vi "Main_09a.vi"() -> ()   [LabVIEW 2020]
uses:
  Point.ctl
panel:
  out "Tail Positon count":i32
  in  "Puzzle":string="R 1\nD 1\nL 1\nD 1\nR 2\nL 1\nU 2\nD 1\nU 2\nL 1\nU 1\nL 2\nD 1\nU 2\nL 1\nR 1\nD 1\nL 2\nD 2\nL 2\nR 1\nL 2\nU 2\nR 2\nL 2\nU 2\nL 1\nD 1\nL 2\nU 1\nR 1\nD 2\nL 2\nU 1\nR 1\nD 1\nU 2\nL 1\nD 2\nU 1\nD 1\nR 2\nD 1\nL 2\nD 1\nL 1\nR 1\nD 2\nL 1\nR 2\nD 2\nU 2\nR 2\nD 2\nR 2\nL 2\nD 2\nL 2\nD 1\nU 2\nR 1\nD 2\nL 2\nR 2\nL 1\nD 1\nU 2\nD 1\nR 2\nU 2\nR 2\nD 1\nL 1\nU 2\nD 1\nU 1\nD 2\nU 1\nR 1\nU 2\nD 1\nL 2\nU 1\nL 2\nD 2\nR 1\nU 2\nL 1\nD 2\nR 1\nU 1\nD 1\nL 2\nU 1\nR 1\nD 2\nU 2\nL 1\nU 2\nD 2\nR 1\nU 2\nR 1\nU 2\nR 1\nD 2\nU 1\nD 2\nL 2\nD 2\nL 2\nD 2\nR 1\nU 1\nD 3\nU 1\nR 2\nU 3\nD 1\nU 2\nD 2\nU 2\nD 1\nU 2\nR 2\nL 2\nU 1\nL 3\nD 1\nR 3\nD 3\nR 2\nL 1\nU 3\nD 1\nU 2\nR 2\nD 1\nR 3\nD 2\nR 3\nD 1\nU 3\nL 3\nR 2\nU 3\nL 3\nU 2\nL 3\nD 1\nR 3\nU 3\nR 2\nD 1\nU 3\nR 3\nD 1\nL 2\nD 2\nL 2\nD 3\nR 2\nU 3\nL 3\nD 2\nU 3\nL 2\nU 3\nD 1\nL 1\nD 3\nR 1\nD 3\nU 1\nL 3\nU 1\nD 2\nU 1\nD 1\nU 2\nD 3\nL 1\nU 1\nR 1\nU 3\nD 3\nR 1\nL 2\nR 3\nL 3\nU 1\nD 2\nR 2\nU 2\nD 3\nU 2\nD 3\nL 1\nR 3\nD 3\nR 2\nU 3\nD 3\nL 2\nR 3\nD 3\nR 2\nL 1\nR 3\nD 2\nR 1\nD 3\nL 1\nU 1\nD 2\nR 1\nD 1\nL 1\nR 2\nL 1\nU 1\nL 2\nD 2\nL 2\nD 1\nL 2\nU 3\nD 1\nR 3\nL 2\nR 1\nL 2\nR 3\nU 2\nL 4\nR 3\nL 1\nR 2\nD 2\nL 4\nU 3\nL 1\nD 1\nL 3\nU 2\nL 3\nU 2\nL 1\nR 2\nL 3\nU 1\nD 2\nR 1\nL 4\nR 4\nL 4\nU 2\nD 2\nR 2\nL 2\nU 2\nR 1\nD 3\nL 4\nR 2\nU 1\nL 4\nR 1\nL 1\nD 4\nR 3\nD 1\nR 2\nL 2\nR 3\nL 1\nU 1\nD 3\nU 2\nR 1\nL 1\nD 3\nR 2\nU 2\nR 3\nU 2\nD 1\nR 4\nU 4\nD 3\nU 3\nR 2\nU 1\nL 1\nU 4\nD 1\nR 4\nD 4\nL 3\nU 4\nR 4\nL 1\nR 1\nU 2\nR 4\nD 2\nR 1\nU 2\nL 1\nD 1\nL 3\nR 3\nL 3\nD 3\nL 4\nD 2\nU 2\nD 3\nR 1\nU 1\nD 3\nU 1\nR 3\nD 2\nL 3\nR 2\nD 1\nL 3\nD 3\nU 3\nD 4\nL 2\nU 3\nD 5\nL 2\nD 2\nR 2\nL 3\nD 5\nU 4\nR 1\nD 5\nR 1\nD 1\nL 2\nR 4\nU 2\nD 3\nR 5\nL 2\nR 2\nD 1\nR 2\nU 5\nL 4\nU 5\nD 1\nL 2\nU 2\nR 2\nD 4\nU 3\nL 2\nD 1\nU 4\nL 4\nD 3\nL 3\nD 3\nR 1\nU 1\nR 1\nU 1\nR 2\nD 3\nR 5\nU 1\nD 2\nL 5\nU 5\nL 4\nD 4\nU 4\nL 1\nR 5\nU 2\nL 3\nU 2\nD 3\nL 5\nD 5\nL 2\nU 2\nD 4\nU 3\nD 3\nL 1\nD 2\nR 2\nD 1\nR 4\nL 3\nD 1\nU 4\nL 1\nR 2\nL 4\nD 5\nR 3\nD 1\nL 5\nD 5\nU 3\nR 2\nD 4\nL 2\nR 2\nD 3\nR 3\nU 2\nR 5\nU 4\nR 3\nL 1\nD 2\nU 1\nL 1\nR 2\nU 4\nD 4\nL 1\nR 1\nU 4\nL 3\nU 5\nR 3\nL 4\nD 3\nU 1\nR 4\nU 1\nL 1\nU 3\nR 4\nL 5\nD 1\nU 4\nR 5\nL 1\nR 4\nD 2\nL 6\nD 5\nU 5\nL 5\nR 6\nD 1\nU 2\nR 1\nU 4\nD 6\nL 6\nD 6\nU 6\nD 4\nU 4\nD 1\nU 3\nL 5\nD 6\nR 1\nL 1\nD 2\nL 4\nD 4\nL 4\nR 4\nU 2\nL 3\nD 4\nR 3\nD 4\nU 5\nR 4\nU 1\nR 6\nL 3\nR 2\nU 1\nL 1\nR 2\nD 3\nR 6\nD 6\nU 1\nD 3\nU 4\nD 5\nL 5\nU 3\nD 6\nL 5\nR 5\nU 1\nR 4\nD 2\nL 2\nR 4\nL 5\nR 4\nL 3\nD 5\nR 6\nL 6\nU 1\nR 5\nU 6\nD 2\nR 2\nD 1\nL 6\nU 4\nL 1\nR 5\nL 1\nR 2\nD 1\nL 4\nU 4\nL 1\nR 3\nU 5\nL 2\nD 6\nU 5\nR 6\nD 6\nU 3\nL 3\nU 3\nL 4\nD 5\nU 2\nD 4\nU 5\nR 6\nU 5\nD 2\nU 6\nD 3\nL 3\nD 6\nL 5\nR 2\nD 6\nR 7\nD 3\nL 7\nD 3\nU 2\nR 7\nU 2\nL 6\nR 7\nD 3\nR 7\nU 5\nR 7\nL 5\nR 7\nL 7\nU 4\nD 4\nU 1\nD 3\nU 1\nD 5\nR 3\nU 1\nD 2\nU 1\nL 4\nU 2\nL 6\nD 7\nU 1\nD 4\nU 6\nL 4\nR 4\nD 4\nR 6\nD 7\nR 1\nD 7\nL 4\nR 4\nL 1\nU 1\nR 6\nL 7\nD 7\nL 5\nU 7\nD 3\nL 6\nD 6\nU 4\nR 1\nL 2\nD 4\nR 3\nL 1\nR 7\nD 1\nL 2\nU 1\nD 2\nR 1\nU 3\nD 4\nL 3\nU 6\nL 4\nR 2\nL 1\nU 6\nD 1\nR 5\nU 2\nD 2\nL 7\nU 2\nR 5\nD 2\nR 4\nD 4\nR 3\nL 2\nR 3\nU 7\nL 5\nR 7\nU 2\nL 7\nD 3\nU 6\nD 4\nU 4\nD 6\nU 3\nL 6\nR 4\nD 2\nR 4\nD 2\nR 3\nL 5\nD 1\nU 7\nD 4\nL 4\nU 2\nD 2\nU 7\nL 5\nR 6\nU 8\nL 7\nD 2\nU 1\nR 6\nD 4\nL 4\nR 7\nD 1\nL 6\nD 7\nR 7\nU 3\nL 6\nU 1\nL 8\nD 6\nU 8\nL 7\nU 5\nD 8\nL 2\nD 3\nL 8\nU 1\nD 5\nL 4\nR 6\nD 8\nL 6\nU 5\nR 3\nU 7\nR 6\nU 3\nL 3\nD 4\nR 4\nL 2\nR 6\nD 3\nR 3\nL 8\nU 2\nD 6\nU 3\nD 8\nU 6\nD 4\nU 8\nR 7\nD 2\nU 6\nD 6\nR 1\nU 3\nD 3\nR 1\nU 3\nR 1\nD 7\nL 8\nR 8\nU 7\nR 3\nL 8\nU 2\nL 8\nD 4\nU 4\nR 1\nD 3\nR 4\nU 3\nL 7\nU 2\nR 7\nD 2\nU 4\nD 3\nL 8\nD 5\nL 3\nU 4\nD 6\nL 5\nD 2\nU 1\nR 6\nL 4\nR 6\nU 5\nR 8\nU 8\nD 7\nL 5\nD 2\nL 8\nU 2\nD 1\nR 1\nL 7\nU 4\nR 2\nU 7\nD 6\nR 6\nL 5\nU 8\nD 7\nR 8\nL 8\nD 6\nU 6\nR 1\nD 5\nL 7\nR 8\nL 4\nD 3\nL 2\nU 5\nR 9\nL 8\nD 8\nL 2\nR 4\nL 7\nR 5\nL 1\nR 8\nD 8\nL 4\nU 2\nD 7\nL 7\nD 6\nR 8\nL 3\nD 7\nU 1\nR 6\nD 6\nU 6\nL 9\nD 1\nR 7\nL 5\nR 5\nU 5\nD 4\nL 8\nU 4\nD 8\nR 4\nD 6\nU 3\nD 7\nL 5\nD 6\nR 9\nU 4\nR 6\nL 3\nU 4\nD 9\nL 7\nR 5\nD 9\nL 6\nU 7\nL 7\nR 4\nD 5\nR 7\nL 5\nR 3\nU 8\nL 6\nU 5\nL 9\nR 8\nU 4\nD 2\nL 4\nD 7\nR 7\nD 4\nL 4\nU 2\nL 3\nR 1\nD 3\nU 6\nR 1\nU 8\nR 2\nL 4\nD 3\nL 5\nU 4\nR 7\nL 2\nR 7\nL 9\nD 9\nU 5\nL 4\nU 1\nD 1\nU 6\nD 1\nL 6\nD 7\nU 5\nD 9\nR 9\nD 5\nU 9\nL 3\nR 5\nD 10\nR 1\nU 7\nD 6\nL 3\nU 5\nR 1\nD 5\nR 8\nU 3\nL 1\nD 2\nR 1\nL 6\nR 8\nD 9\nU 9\nD 4\nR 1\nU 8\nL 5\nU 4\nD 7\nL 1\nR 4\nL 6\nD 4\nR 5\nD 1\nR 10\nD 5\nR 7\nU 6\nR 5\nU 2\nL 8\nR 1\nU 3\nL 5\nU 4\nL 3\nD 3\nU 6\nD 10\nL 3\nD 7\nL 5\nD 4\nU 6\nR 9\nU 5\nD 5\nR 2\nL 7\nU 8\nD 5\nR 9\nL 6\nR 8\nU 9\nL 4\nR 10\nD 10\nL 9\nR 8\nL 4\nR 5\nL 9\nD 1\nL 3\nR 9\nU 2\nL 5\nR 2\nU 1\nR 4\nD 10\nU 3\nD 8\nL 9\nD 8\nL 5\nD 4\nU 2\nL 8\nR 5\nU 4\nD 1\nL 4\nU 7\nD 9\nR 3\nD 7\nR 9\nL 6\nR 6\nU 8\nL 10\nU 5\nD 4\nR 5\nL 6\nD 7\nL 10\nR 1\nL 9\nU 6\nD 9\nR 7\nL 7\nD 6\nU 6\nR 1\nD 7\nL 1\nR 9\nD 9\nR 3\nL 5\nD 4\nR 3\nL 5\nD 11\nU 1\nR 6\nD 8\nR 4\nD 3\nR 9\nU 3\nD 8\nU 7\nR 2\nU 10\nR 4\nL 4\nD 10\nR 8\nU 11\nR 7\nD 7\nR 9\nD 11\nU 6\nR 7\nD 10\nL 4\nD 5\nL 7\nD 3\nL 4\nD 4\nU 4\nR 3\nL 9\nD 4\nL 8\nU 5\nR 7\nL 2\nD 4\nR 11\nU 10\nD 3\nR 8\nD 3\nR 10\nL 8\nU 6\nR 4\nD 10\nR 7\nD 3\nR 2\nU 1\nD 5\nL 8\nU 2\nR 1\nU 8\nR 11\nL 3\nU 10\nL 5\nD 3\nL 6\nU 10\nL 11\nD 4\nL 5\nD 1\nL 4\nD 1\nL 3\nR 7\nU 7\nR 4\nL 1\nU 10\nD 11\nL 1\nR 1\nU 9\nD 6\nL 9\nD 1\nL 4\nD 11\nL 5\nU 2\nL 5\nD 8\nU 10\nD 5\nU 10\nL 8\nR 11\nD 10\nU 11\nR 4\nU 6\nD 11\nR 1\nL 4\nU 12\nL 8\nU 12\nD 4\nL 7\nU 7\nL 8\nD 3\nU 1\nL 12\nD 5\nU 3\nD 6\nR 7\nU 1\nD 12\nR 6\nU 3\nD 3\nR 12\nU 5\nR 3\nU 8\nL 6\nR 6\nU 3\nL 4\nD 8\nL 5\nD 12\nU 1\nL 9\nR 4\nL 1\nD 6\nU 9\nL 5\nR 3\nL 9\nD 8\nR 6\nD 3\nU 6\nL 1\nD 7\nU 5\nD 1\nL 11\nR 7\nD 11\nL 3\nU 6\nR 9\nD 12\nR 11\nL 5\nR 8\nL 2\nU 10\nR 6\nU 10\nL 9\nU 1\nL 1\nR 8\nL 7\nR 3\nU 4\nL 3\nR 8\nL 9\nR 11\nL 9\nD 11\nU 1\nL 12\nR 6\nL 3\nR 3\nD 12\nU 9\nL 9\nD 8\nR 4\nL 7\nR 1\nU 2\nR 4\nU 4\nR 11\nU 7\nD 11\nU 3\nD 6\nU 7\nL 2\nD 4\nU 9\nR 3\nL 8\nR 9\nL 4\nR 5\nL 7\nD 3\nR 8\nL 6\nU 10\nR 3\nL 6\nD 8\nU 3\nD 9\nL 1\nU 13\nR 12\nL 13\nR 2\nU 8\nR 1\nD 11\nR 5\nL 4\nU 5\nL 3\nD 13\nU 2\nD 1\nU 2\nL 9\nD 3\nR 6\nU 13\nL 3\nU 5\nR 2\nD 2\nL 5\nU 4\nR 6\nD 1\nU 9\nL 7\nR 11\nU 10\nD 12\nR 10\nU 7\nR 5\nL 2\nR 13\nL 13\nD 3\nR 7\nU 1\nL 1\nD 2\nL 9\nU 12\nD 7\nU 13\nL 12\nU 13\nD 7\nU 7\nD 8\nL 2\nU 6\nD 2\nU 6\nL 8\nU 4\nD 11\nU 11\nL 11\nR 10\nL 10\nR 6\nD 13\nU 2\nL 7\nU 8\nD 1\nR 6\nL 7\nR 9\nL 8\nR 9\nL 6\nR 7\nD 12\nR 11\nL 8\nR 1\nD 5\nR 5\nL 10\nU 6\nL 8\nD 9\nL 5\nU 4\nD 12\nU 8\nL 13\nU 6\nD 10\nR 5\nL 13\nD 7\nL 13\nR 5\nL 10\nD 13\nL 9\nR 3\nD 8\nU 9\nD 10\nU 10\nD 7\nL 5\nR 5\nD 9\nL 7\nR 10\nD 13\nR 1\nU 2\nR 6\nU 14\nR 10\nD 6\nU 13\nD 14\nU 5\nD 1\nU 8\nR 4\nU 9\nR 13\nL 4\nD 2\nR 8\nU 2\nD 12\nU 3\nR 6\nU 6\nD 11\nR 7\nL 12\nR 9\nU 7\nD 1\nR 14\nL 11\nU 4\nD 13\nU 5\nL 7\nR 14\nL 1\nU 6\nD 3\nL 1\nU 13\nD 8\nU 14\nD 5\nU 14\nL 1\nR 1\nD 5\nU 7\nL 8\nR 6\nU 1\nD 2\nR 14\nU 13\nL 10\nU 8\nD 13\nU 6\nR 2\nD 4\nR 6\nU 7\nD 10\nL 6\nU 5\nL 3\nD 9\nU 13\nD 8\nU 3\nR 3\nL 12\nD 5\nR 8\nU 7\nR 11\nU 6\nD 7\nR 13\nU 1\nD 9\nU 10\nD 3\nL 5\nR 12\nL 4\nD 13\nR 7\nD 12\nR 11\nD 9\nR 5\nU 13\nR 3\nD 4\nU 10\nR 3\nU 6\nL 4\nR 1\nU 4\nL 9\nD 11\nU 5\nD 3\nU 13\nD 1\nL 1\nD 13\nL 2\nR 9\nL 4\nR 2\nU 9\nD 9\nU 12\nL 14\nR 2\nL 9\nR 5\nU 2\nD 3\nR 13\nU 5\nD 1\nU 15\nR 6\nD 14\nR 8\nL 9\nD 14\nL 6\nR 8\nU 14\nR 11\nL 3\nD 15\nU 5\nR 1\nL 7\nR 12\nD 1\nR 4\nD 13\nU 9\nD 2\nL 3\nU 10\nR 10\nD 2\nR 6\nU 13\nD 7\nR 5\nU 5\nL 12\nU 6\nR 1\nL 7\nU 9\nD 15\nL 8\nU 9\nL 5\nR 3\nL 9\nU 6\nL 11\nD 8\nL 11\nD 13\nU 3\nR 6\nD 2\nL 10\nR 15\nU 2\nD 8\nR 6\nD 6\nL 8\nD 7\nU 2\nD 14\nU 4\nR 6\nD 15\nL 12\nR 4\nD 3\nU 7\nD 10\nL 8\nU 7\nR 10\nU 11\nD 2\nR 10\nD 10\nU 13\nR 8\nL 2\nU 12\nR 9\nU 12\nR 5\nU 10\nL 6\nR 3\nD 10\nL 10\nU 6\nL 4\nR 3\nD 9\nR 15\nD 14\nL 11\nR 5\nU 2\nR 14\nL 15\nR 3\nD 3\nL 4\nU 10\nD 14\nL 9\nD 5\nL 16\nU 12\nL 4\nD 15\nL 10\nR 14\nD 4\nR 12\nL 7\nU 5\nR 3\nL 6\nU 16\nL 5\nU 8\nD 8\nL 6\nD 3\nU 14\nR 1\nL 13\nU 4\nD 11\nR 5\nL 11\nD 7\nR 1\nL 14\nU 10\nL 5\nD 15\nU 14\nL 4\nD 7\nU 3\nR 1\nU 2\nR 3\nD 16\nU 7\nR 7\nD 13\nR 7\nD 5\nU 7\nR 16\nU 4\nL 3\nR 9\nU 1\nD 2\nR 5\nD 3\nU 8\nR 5\nL 13\nU 13\nL 2\nR 9\nL 14\nD 10\nR 1\nU 1\nR 14\nU 14\nR 2\nL 1\nR 12\nL 1\nD 6\nR 2\nD 7\nR 11\nL 5\nD 8\nR 15\nD 12\nR 12\nL 8\nD 10\nR 2\nD 12\nU 15\nL 9\nD 4\nU 3\nL 8\nD 3\nU 9\nD 16\nL 2\nU 14\nR 15\nD 14\nU 12\nD 6\nU 14\nR 11\nD 12\nR 2\nU 13\nL 2\nR 1\nD 6\nU 13\nD 15\nU 1\nR 14\nL 16\nD 8\nR 13\nL 14\nR 3\nD 8\nL 6\nR 16\nD 6\nL 13\nR 2\nL 11\nD 2\nU 1\nR 15\nL 9\nU 1\nR 12\nL 9\nD 7\nL 8\nU 2\nL 14\nR 7\nU 8\nD 15\nR 8\nD 13\nL 15\nR 11\nD 17\nU 2\nR 14\nL 9\nU 11\nD 6\nU 4\nD 8\nU 16\nD 5\nL 3\nD 11\nL 7\nU 11\nL 4\nD 5\nL 5\nD 2\nU 8\nR 17\nD 17\nU 12\nR 4\nL 13\nR 15\nL 10\nU 2\nL 10\nR 6\nD 1\nU 6\nL 3\nD 8\nR 4\nD 1\nL 4\nD 13\nR 1\nU 3\nL 1\nU 9\nD 13\nU 2\nD 13\nR 6\nD 8\nR 6\nD 13\nR 4\nD 10\nL 10\nU 8\nD 1\nR 6\nU 14\nR 3\nL 10\nU 15\nL 11\nU 13\nL 4\nU 5\nL 16\nR 16\nU 11\nR 14\nD 7\nU 5\nR 9\nL 5\nU 12\nR 16\nU 10\nD 5\nR 17\nL 3\nD 5\nU 13\nR 3\nU 3\nL 14\nU 1\nL 8\nR 2\nD 3\nU 9\nD 7\nL 1\nD 5\nR 16\nD 12\nR 1\nU 2\nL 16\nU 3\nR 18\nD 11\nR 3\nL 17\nR 7\nL 6\nD 13\nL 5\nR 12\nD 3\nU 1\nL 1\nU 5\nL 8\nR 11\nL 13\nD 14\nR 17\nD 17\nL 2\nU 7\nD 18\nR 3\nD 2\nU 6\nD 9\nR 3\nU 3\nR 5\nD 16\nR 9\nD 13\nU 8\nD 17\nR 4\nL 6\nR 7\nD 2\nR 15\nU 10\nR 15\nD 6\nL 8\nR 17\nD 5\nL 9\nU 18\nD 10\nU 3\nL 6\nU 10\nD 10\nU 16\nR 6\nD 18\nU 10\nD 8\nU 14\nR 3\nU 14\nL 16\nR 3\nD 5\nL 2\nR 4\nD 9\nL 13\nR 17\nL 8\nD 2\nR 16\nD 18\nL 11\nD 15\nU 5\nD 7\nU 14\nD 13\nU 7\nL 13\nD 13\nR 1\nD 15\nR 11\nL 1\nU 6\nD 14\nL 6\nU 8\nD 15\nR 8\nL 12\nD 17\nR 8\nL 17\nD 16\nR 9\nD 19\nU 4\nR 9\nU 10\nL 3\nU 3\nD 5\nR 2\nU 6\nL 16\nD 8\nR 4\nL 16\nR 15\nU 6\nL 8\nD 6\nL 6\nR 1\nL 8\nD 13\nL 1\nU 7\nR 16\nL 16\nU 1\nL 18\nD 16\nL 8\nU 2\nD 1\nR 2\nD 10\nU 8\nD 2\nR 18\nU 14\nD 15\nR 15\nU 3\nD 1\nU 17\nL 17\nD 15\nL 14\nR 6\nL 18\nU 19\nL 6\nU 17\nL 1\nD 2\nU 17\nR 11\nL 3\nR 3\nL 12\nU 1\nL 9\nU 13\nD 15\nU 12\nR 1\nL 5\nD 17\nL 14\nD 13\nL 2\nD 10\nU 5\nR 13\nL 19\nD 1\nR 12\nU 17\nR 15\nD 19\nU 12\nD 16\nR 2\nU 3\nR 15\nL 13\nU 11\nD 19\nR 10\nD 19\nL 2\nU 12\nR 5\nL 13\nU 13\nR 1\nD 11\nR 17\nD 7\nU 4\nD 14\nL 13\nR 8\nL 8\nD 8"
  in  "Example":string="R 4\nU 4\nL 3\nD 1\nR 4\nD 1\nL 5\nR 2"
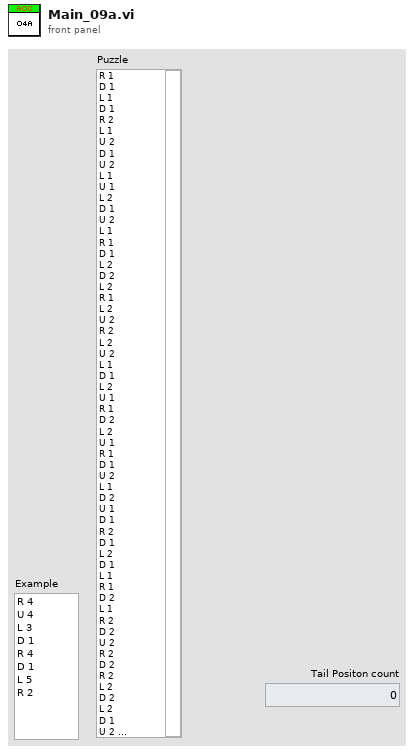
[diagram p1: front panel]
types:
  T1 = typedef "Point.ctl" = cluster{"X":i32, "Y":i32}
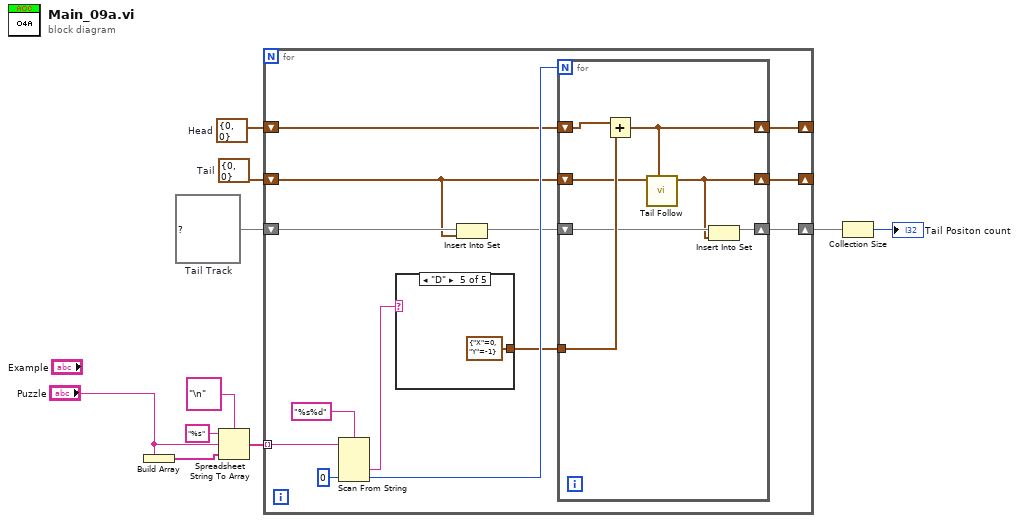
[diagram p0: block diagram]
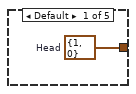
[diagram p2: hidden frame]
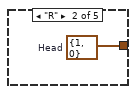
[diagram p3: hidden frame]
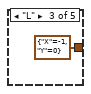
[diagram p4: hidden frame]
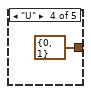
[diagram p5: hidden frame]
diagram:
  w6 = set{T1} {}  # Tail Track
  w5 = T1 {"X"=0, "Y"=0}  # Tail
  w4 = T1 {"X"=0, "Y"=0}  # Head
  n1 = Build Array("Puzzle") -> (w10:string[])
  n2 = Spreadsheet String To Array(delimiter (Tab)="\n", format string="%s", spreadsheet string="Puzzle", array type (2D Dbl)=w10) -> (array=w7:string[])
  n3 = for {
    tunnel: w7 -> [w22] mode=indexing
    shift-right: [w17] -> _
    shift-left: w4 -> [w18]
    shift-right: [w16] -> _
    shift-left: w5 -> [w11]
    shift-right: [w15] -> w3
    shift-left: w6 -> [w13]
    n4 = Scan From String(format string="%s%d", input string=w22, default 2=0 ("default value 2")) -> (output 1=w21:string, output 2=w19:i32)  [unwired: 3 in, 3 out]
    n5 = case shown="\"D\"" w21 {
      tunnel: [w31 w32 T1 {"X"=-1, "Y"=0} ("Head") T1 {"X"=0, "Y"=1} ("Head") T1 {"X"=0, "Y"=-1} ("Head")] -> w14
      frame Default {
        w31 = T1 {"X"=1, "Y"=0}  # Head
      }
      frame "R" {
        w32 = T1 {"X"=1, "Y"=0}  # Head
      }
      frame "L" {
      }
      frame "U" {
      }
      frame "D" {
      }
    }
    n6 = Insert Into Set(10:w11, 11:w13) -> (3:w12:set{T1})  [unwired: 1 out]
    n7 = for {
      N: w19 -> [_]
      shift-right: [w25] -> w17
      shift-left: w18 -> [w30]
      shift-right: [w26] -> w16
      shift-left: w11 -> [w24]
      shift-right: [w27] -> w15
      shift-left: w12 -> [w28]
      tunnel: w14 -> [w29]
      n8 = Add(x=w30, y=w29) -> (x+y=w25:T1)
      n9 = call "Tail Follow.vi"("Head"=w25, "Tail"=w24) -> ("Tail Out"=w26:T1)  [unwired: 9 in]
      n10 = Insert Into Set(10:w26, 11:w28) -> (3:w27:set{T1})  [unwired: 1 out]
    }
  }
  n11 = Collection Size(1:w3) -> (0:→"Tail Positon count":i32)
